vi "RSNRPZ Set Scope Terminal Control.vi"(8 "error in (no error)":errorcluster, 9 "Terminal Control (1: Repeat)":i32(ring)=1 items=["Moving", "Repeat"], 10 "Channel (1)":i32=1, 11 "VISA session":refnum<visa-resource-name> caption="VISA resource name") -> (0 "error out":errorcluster, 3 "dup VISA session":refnum<visa-resource-name> caption="VISA resource name")   [LabVIEW 2010]
doc: "As soon as a new single value is determined, the filter window is advanced by one value so that the new value is taken into account by the filter and the oldest value is forgotten.\nTerminal control then determines in the Scope mode whether a new result will be calculated immediately after a new measured value is available or only after an entire range of new values is available for the filter.\n\nNote:\n\n1) This VI is not available for NRP-Z51.\n\nRemote-control command(s):\nSENS:TRAC:AVER:TCON MOV | REP"
uses:
  rsnrpz_32.dll
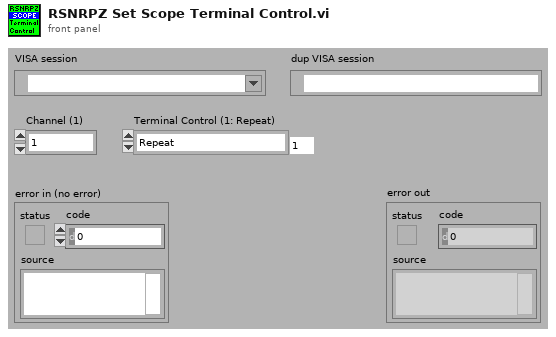
[diagram p1: front panel]
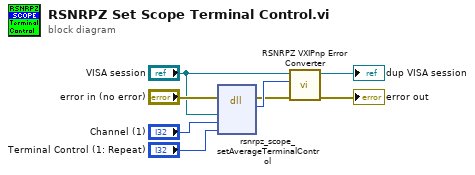
[diagram p0: block diagram]
diagram:
  n1 = dll-call lib="rsnrpz_32.dll" fn="rsnrpz_scope_setAverageTerminalControl"(error in="error in (no error)", "VISA Session"="VISA session", "Channel"="Channel (1)", "Terminal Control"="Terminal Control (1: Repeat)") -> (error out=w5:errorcluster, "Status"=w8:i32)  [unwired: 5 in, 1 out]
  n2 = call <instrlib>:"RSNRPZ VXIPnp Error Converter.vi"("error in"=w5, "VXIPnp error code"=w8, "VISA session"="VISA session") -> ("error out"=→"error out":errorcluster, "dup VISA session"=→"dup VISA session":refnum<visa-resource-name>)  [unwired: 7 in]
